vi "sv_UFF58 Set Record Fields (Freq).vi"(0 "ID lines (1-3)":T9, 4 "spectrum info":T3 {"x-axis units" items=["Time (s)"=0, "Frequency-CB (Hz)"=1, "Frequency-CPB (Hz)"=1248, "Frequency-Arbitrary (Hz)"=2357, "Quefrency (s)"=2, "Revolutions (rev)"=3, "Order"=4, "Speed (RPM)"=11, "Speed (rad/s)"=21, "Index"=65535]; "weighting filter" items=["Linear", "A-weighting", "B-weighting", "C-weighting", "ITU-R 468-4", "Dolby", "CCITT", "C-message", "Wb", "Wc", "Wd", "We", "Wf", "Wh", "Wj", "Wk", "Wm", "AES17 20 kHz lowpass", "AES17 40 kHz lowpass", "AES17 20 kHz highpass", "AES17 40 kHz highpass"]; "dB reference [EU]" format="%.2f"; "engineering units" items=["custom..."=0, "V"=1, "A"=21, "C"=30, "pC"=31, "s"=32, "-"=29, "Pa"=2, "N"=20, "g"=3, "m/s^2"=4, "m/s"=5, "m"=6, "mm/s"=12, "mm"=13, "micron/s"=14, "micron"=15, "in/s^2"=7, "in/s"=8, "in"=9, "mil/s"=10, "mil"=11, "rad/s^2"=16, "rad/s"=17, "rad"=18, "deg/s^2"=26, "deg/s"=27, "deg"=28, "RPM"=22, "cycle/s^2"=23, "Hz"=24, "cycle"=25, "strain"=19]; "spectral info"."window" items=["None "=0, "Hanning"=1, "Hamming"=2, "Blackman-Harris"=3, "Exact Blackman"=4, "Blackman"=5, "Flat Top"=6, "4 Term B-Harris "=7, "7 Term B-Harris"=8, "Low Sidelobe"=9, "Force - Exponential"=10, "Gaussian"=62]}, 5 "error in (no error)":errorcluster) -> (7 "DOF identification (record 6)":T10 {"reference direction" items=["-Z Rotation"=-6, "-Y Rotation"=-5, "-X Rotation"=-4, "-Z Translation"=-3, "-Y Translation"=-2, "-X Translation"=-1, "Scalar"=0, "+X Translation"=1, "+Y Translation"=2, "+Z Translation"=3, "+X Rotation"=4, "+Y Rotation"=5, "+Z Rotation"=6]; "response direction" items=["-Z Rotation"=-6, "-Y Rotation"=-5, "-X Rotation"=-4, "-Z Translation"=-3, "-Y Translation"=-2, "-X Translation"=-1, "Scalar"=0, "+X Translation"=1, "+Y Translation"=2, "+Z Translation"=3, "+X Rotation"=4, "+Y Rotation"=5, "+Z Rotation"=6]}, 9 "abscissa data characteristics (record 8)":T1 {"specific data type" items=["unknown"=0, "general"=1, "stress"=2, "strain"=3, "temperature"=5, "heat flux"=6, "displacement"=8, "reaction force"=9, "velocity"=11, "acceleration"=12, "excitation force"=13, "pressure"=15, "mass"=16, "time"=17, "frequency"=18, "rpm"=19, "order"=20, "sound pressure"=21, "sound intensity"=22, "sound power"=23]}, 11 "ordinate numerator data characteristics (record 9)":T1 {"specific data type" items=["unknown"=0, "general"=1, "stress"=2, "strain"=3, "temperature"=5, "heat flux"=6, "displacement"=8, "reaction force"=9, "velocity"=11, "acceleration"=12, "excitation force"=13, "pressure"=15, "mass"=16, "time"=17, "frequency"=18, "rpm"=19, "order"=20, "sound pressure"=21, "sound intensity"=22, "sound power"=23]}, 12 "ID lines (1-3) out":T9, 13 "ordinate denominator data characteristics (record 10)":T1 {"specific data type" items=["unknown"=0, "general"=1, "stress"=2, "strain"=3, "temperature"=5, "heat flux"=6, "displacement"=8, "reaction force"=9, "velocity"=11, "acceleration"=12, "excitation force"=13, "pressure"=15, "mass"=16, "time"=17, "frequency"=18, "rpm"=19, "order"=20, "sound pressure"=21, "sound intensity"=22, "sound power"=23]}, 19 "error out":errorcluster)   [LabVIEW 2017, in "SoundVib_UFF58.lvlib"]
doc: "This VI sets the following record values:\nRecords (1-3) (name): <B>ID lines (1-3) out</B>\nRecord 6 (function type): <B>DOF identification (record 6)</B>\nRecord 8 (specific data type, axis label, unit label): <B>abscissa data characteristics (record 8)</B>\nRecord 9 (specific data type, axis label, unit label): <B>ordinate numerator data characteristics (record 9)</B>\nRecord 10 (specific data type, axis label, unit label): <B>ordinate denominator data characteristics (record 10)</B>"
uses:
  <vilib>/addons/Sound and Vibration/svt_UFF58/SoundVib_UFF58.lvlib
  <vilib>/addons/Sound and Vibration/svt_UFF58/subVIs/sv_UFF58 Axis Characteristics.ctl
  <vilib>/addons/Sound and Vibration/svt_UFF58/subVIs/sv_UFF58 Specific Datatype.ctl
  <vilib>/addons/Sound and Vibration/svt_UFF58/subVIs/sv_UFF58 DOF.ctl
  <vilib>/addons/Sound and Vibration/svt_UFF58/subVIs/sv_FunctionType.ctl
  <vilib>/addons/Sound and Vibration/svt_UFF58/subVIs/sv_UFF58 Response Direction.ctl
  <vilib>/addons/Sound and Vibration/svt_UFF58/subVIs/sv_IDLines123.ctl
  <vilib>/addons/_NISVFA/_Shared subVIs/Controls/svc_Spectrum Info.ctl
  <vilib>/addons/_NISVFA/_Shared subVIs/Controls/svc_X-Axis Units.ctl
  <vilib>/addons/_NISVFA/_Shared subVIs/Controls/svc_Spectrum Type.ctl
  <vilib>/addons/_NISVFA/_Shared subVIs/Controls/svc_Engineering Units Text Ring.ctl
  <vilib>/addons/_NISVFA/_Shared subVIs/Controls/svc_Weighting Filter Text Ring.ctl
  <vilib>/addons/_NISVFA/_Shared subVIs/Controls/svc_Complimentary Spectrum Units.ctl
  <vilib>/addons/_NISVFA/_Shared subVIs/Common/svc_Get Weighting Enum and Labels.vi
  <vilib>/addons/_NISVFA/_Shared subVIs/Common/svc_Unit Label Lexical Class.vi
  <vilib>/addons/_NISVFA/_Shared subVIs/Common/svc_Engineering Units to Unit Label.vi
  <vilib>/addons/_NISVFA/_Shared subVIs/Common/svc_Format Value (DBL).vi
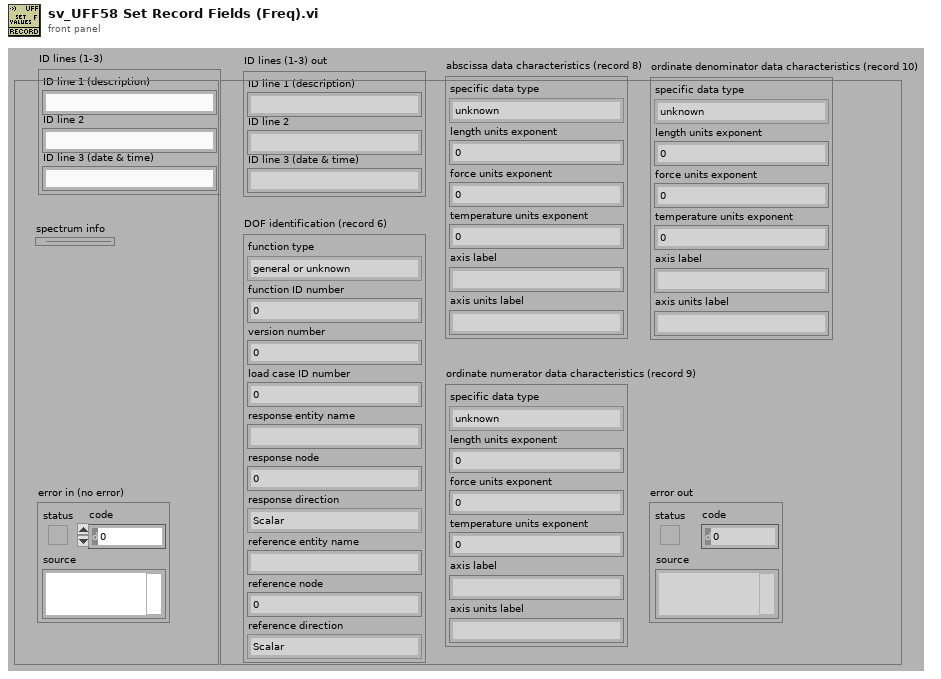
[diagram p1: front panel]
types:
  T1 = typedef "SoundVib_UFF58.lvlib/sv_UFF58 Axis Characteristics.ctl" = cluster{"specific data type":T2, "length units exponent":i32, "force units exponent":i32, "temperature units exponent":i32, "axis label":string, "axis units label":string}
  T2 = typedef "SoundVib_UFF58.lvlib/sv_UFF58 Specific Datatype.ctl" = u16
  T3 = typedef "svc_Spectrum Info.ctl" = cluster{"channel name":string, "description":string, "x-axis units":T4, "spectral info":cluster{"spectrum type":T5, "linear/dB":enum16{"linear", "dB"}, "window":u16, "window size":i32, "FFT size":i32}, "engineering units":T6, "custom label":string, "dB reference [EU]":dbl, "peak units":enum16{"rms", "peak", "peak-peak"}, "weighting filter":T7, "spectral density?":bool, "unit label":string, "spectrum skewed?":bool, "complimentary spectrum units":T8}
  T4 = typedef "svc_X-Axis Units.ctl" = u16
  T5 = typedef "svc_Spectrum Type.ctl" = enum16{"FFT Spectrum [complex]", "Amplitude [Magnitude]", "Power [Magnitude^2]", "Cross Spectrum [complex]", "Frequency Response [Complex]"}
  T6 = typedef "svc_Engineering Units Text Ring.ctl" = u16
  T7 = typedef "svc_Weighting Filter Text Ring.ctl" = u16
  T8 = typedef "svc_Complimentary Spectrum Units.ctl" = enum16{"none", "radians", "degrees", "cycles", "imaginary"}
  T9 = typedef "SoundVib_UFF58.lvlib/sv_IDLines123.ctl" = cluster{"ID line 1 (description)":string, "ID line 2":string, "ID line 3 (date & time)":string}
  T10 = typedef "SoundVib_UFF58.lvlib/sv_UFF58 DOF.ctl" = cluster{"function type":T11, "function ID number":i32, "version number":i32, "load case ID number":i32, "response entity name":string, "response node":i32, "response direction":T12, "reference entity name":string, "reference node":i32, "reference direction":T12}
  T11 = typedef "SoundVib_UFF58.lvlib/sv_FunctionType.ctl" = enum16{"general or unknown", "time response", "auto spectrum", "cross spectrum", "frequency response function", "transmissibility", "coherence", "auto correlation", "cross correlation", "power spectral density (PSD)", "energy spectral density (ESD)", "probability density function", "spectrum", "cumulative frequency distribution", "peaks valley", "stress/cycles", "strain/cycles", "orbit", "mode indicator function", "force pattern", "partial power", "partial coherence", "eigenvalue", "eigenvector", "shock response spectrum", "finite impulse response filter", "multiple coherence", "order function", "phase compensation"}
  T12 = typedef "SoundVib_UFF58.lvlib/sv_UFF58 Response Direction.ctl" = i32
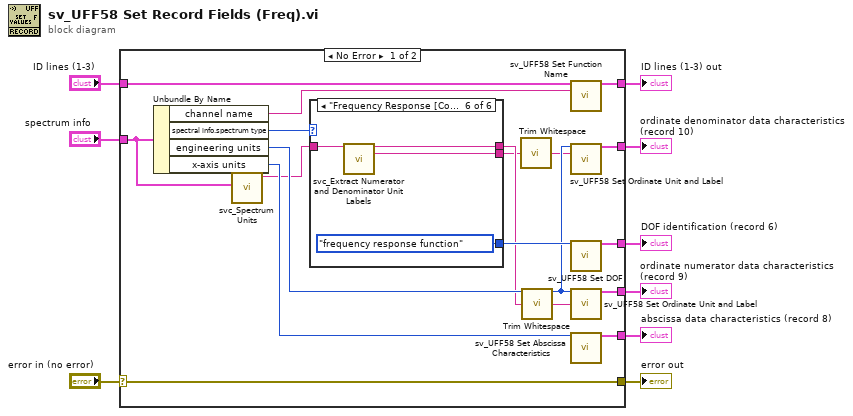
[diagram p0: block diagram]
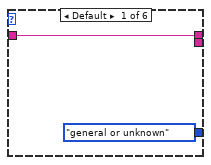
[diagram p2: hidden frame]
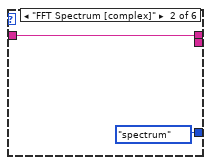
[diagram p3: hidden frame]
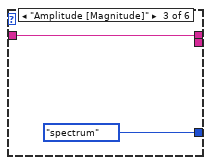
[diagram p4: hidden frame]
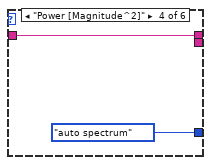
[diagram p5: hidden frame]
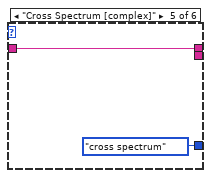
[diagram p6: hidden frame]
diagram:
  n1 = case shown="No Error" "error in (no error)" {
    selector: "error in (no error)" -> [w19 w43]
    tunnel: [w27 _] -> w9
    tunnel: [w26 _] -> w8
    tunnel: [w25 w42] -> w7
    tunnel: "ID lines (1-3)" -> [w24 w42]
    tunnel: [w23 _] -> w5
    tunnel: [w22 _] -> w4
    tunnel: "spectrum info" -> [w13 _]
    tunnel: [w19 w43] -> w2
    frame No Error {
      n2 = Unbundle By Name(w13) -> ("channel name"=w15:string, "spectral info.spectrum type"=w21:T5, "engineering units"=w18:T6, "x-axis units"=w14:T4)
      n3 = call <vilib>:"svc_Spectrum Units.vi"("spectrum info in"=w13) -> ("unit label"=w12:string)  [unwired: 3 in, 3 out]
      n4 = case shown="\"Frequency Response [Complex]\"" w21 {
        tunnel: [sv_FunctionType."general or unknown" ("FunctionType") sv_FunctionType."spectrum" ("FunctionType") sv_FunctionType."spectrum" ("FunctionType") sv_FunctionType."auto spectrum" ("FunctionType") sv_FunctionType."cross spectrum" ("FunctionType") sv_FunctionType."frequency response function" ("FunctionType")] -> w20
        tunnel: w12 -> [w28 w30 w32 w34 w36 w40]
        tunnel: [w28 w30 w32 w34 w36 w39] -> w17
        tunnel: [_ _ _ _ _ w38] -> w16
        frame Default {
        }
        frame "FFT Spectrum [complex]" {
        }
        frame "Amplitude [Magnitude]" {
        }
        frame "Power [Magnitude^2]" {
        }
        frame "Cross Spectrum [complex]" {
        }
        frame "Frequency Response [Complex]" {
          n5 = call <vilib>:"svc_Extract Numerator and Denominator Unit Labels.vi"("unit label"=w40) -> ("numerator unit label"=w39:string, "denominator unit label"=w38:string)  [unwired: 13 in]
        }
      }
      n6 = call <vilib>:"Trim Whitespace.vi"("string"=w16) -> ("trimmed string"=w11:string)  [unwired: 1 in]
      n7 = call <vilib>:"Trim Whitespace.vi"("string"=w17) -> ("trimmed string"=w10:string)  [unwired: 1 in]
      n8 = call <vilib>:"sv_UFF58 Set Function Name.vi"("ID lines (1-3) in"=w24, "channel name"=w15) -> ("ID lines (1-3) out"=w25:T9)  [unwired: 12 in, 1 out]
      n9 = call <vilib>:"sv_UFF58 Set Ordinate Unit and Label.vi"("engineering units"=w18, "unit label"=w11) -> ("ordinate data characteristics (record 9 or 10)"=w22:T1)  [unwired: 13 in]
      n10 = call <vilib>:"sv_UFF58 Set DOF.vi"("function type"=w20) -> ("DOF identification (record 6)"=w26:T10)  [unwired: 14 in]
      n11 = call <vilib>:"sv_UFF58 Set Ordinate Unit and Label.vi"("engineering units"=w18, "unit label"=w10) -> ("ordinate data characteristics (record 9 or 10)"=w23:T1)  [unwired: 13 in]
      n12 = call <vilib>:"sv_UFF58 Set Abscissa Characteristics.vi"("x-axis units"=w14) -> ("abscissa data characteristics (record 8)"=w27:T1)  [unwired: 14 in]
    }
    frame Error {
    }
  }
  "abscissa data characteristics (record 8)" <- w9
  "DOF identification (record 6)" <- w8
  "ID lines (1-3) out" <- w7
  "ordinate numerator data characteristics (record 9)" <- w5
  "ordinate denominator data characteristics (record 10)" <- w4
  "error out" <- w2
